vi "Register State.vi"() -> ()   [LabVIEW 2017]
uses:
  user.lib/_NEVSTOP/Communicable State Machine(CSM)/AdvanceAPI/CSM - Revert Arguments-Safe String.vi
  user.lib/_NEVSTOP/Communicable State Machine(CSM)/AdvanceAPI/CSM - Make String Arguments Safe.vi
  user.lib/_NEVSTOP/Communicable State Machine(CSM)/AdvanceAPI/CSM - Break Down Multiple States String.vi
  user.lib/_NEVSTOP/Communicable State Machine(CSM)/AdvanceAPI/CSM - Compact Multiple States.vi
  user.lib/_NEVSTOP/Communicable State Machine(CSM)/AdvanceAPI/CSM - Keywords.vi
  user.lib/_NEVSTOP/Communicable State Machine(CSM)/_Shared/Trim Single-line Text.vi
  user.lib/_NEVSTOP/Communicable State Machine(CSM)/Communicable State Machine.lvlib
panel:
  in  "API: API2 -@submodule2":bool
  in  "API: API1 -@submodule1":bool
  out "State History":string
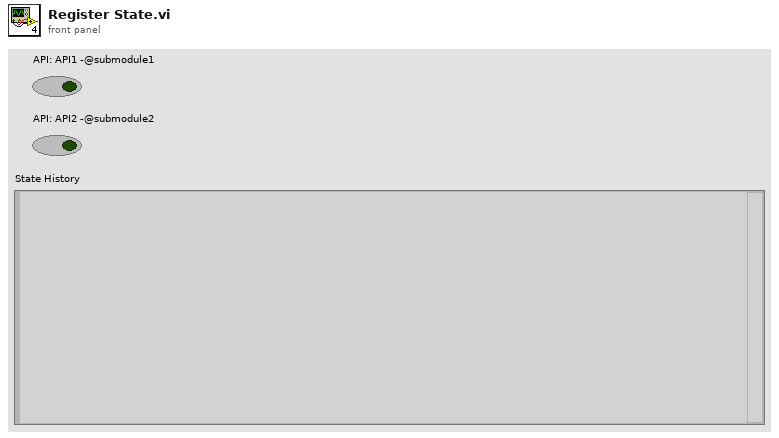
[diagram p1: front panel]
types:
  T1 = enum32{"Invalid", "Standard", "Closed", "Hidden", "Minimized", "Maximized"}
  T2 = enum32{"invalid app kind", "Development System", "Run Time System", "Student Edition", "Embedded LabVIEW", "Evaluation", "Custom"}
  T3 = typedef "Communicable State Machine.lvlib/_CSM_Response Source Message.ctl" = cluster{"‘State":string, "’Arguments":string, "’Error":errorcluster}
  T4 = cluster{"Current VI Reference":refnum<vi>, "Close Panel on Exit?":bool}
  T5 = cluster{"Core":cluster{"Current VI Reference":refnum<vi>, "Close Panel on Exit?":bool}, "Your Boolean data":bool, "Your string data":string}
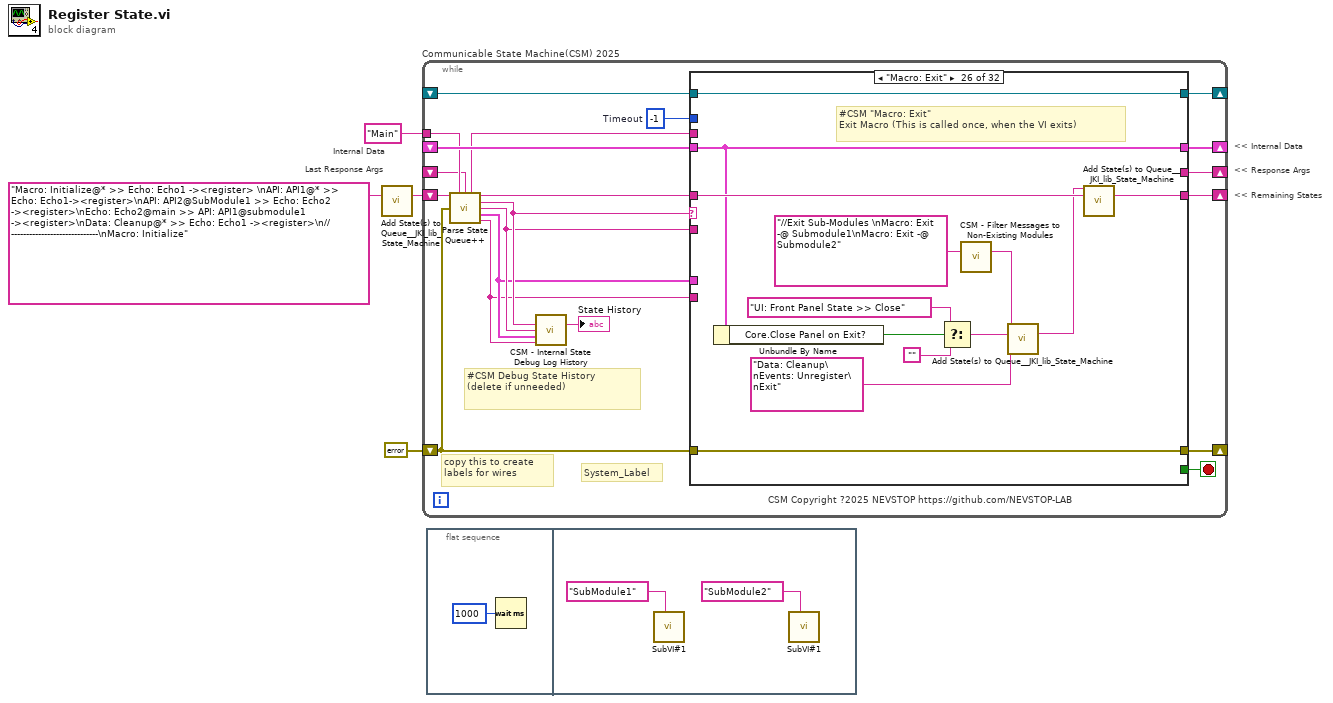
[diagram p0: block diagram]
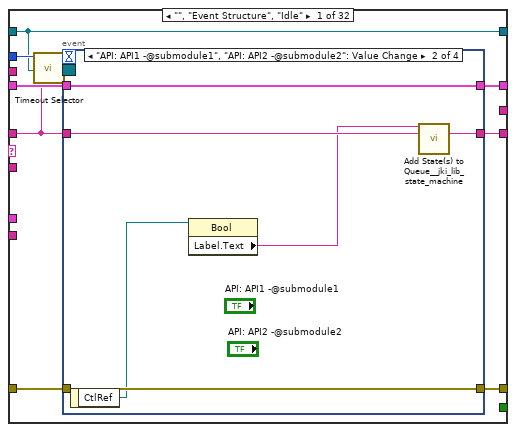
[diagram p2: hidden frame]
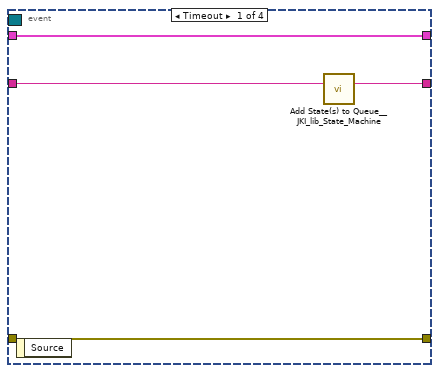
[diagram p3: hidden frame]
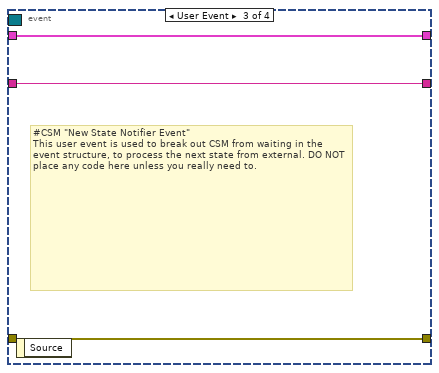
[diagram p4: hidden frame]
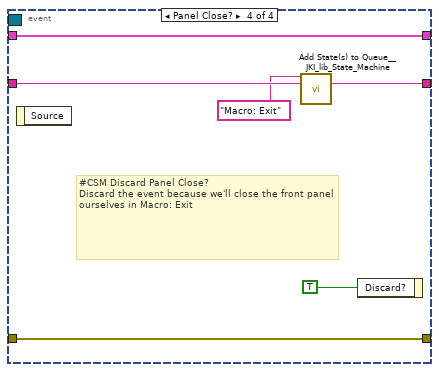
[diagram p5: hidden frame]
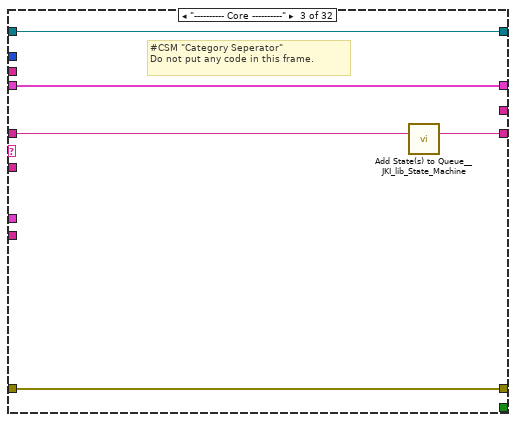
[diagram p7: hidden frame]
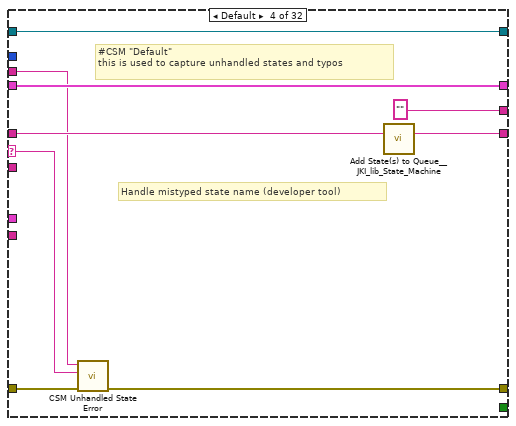
[diagram p8: hidden frame]
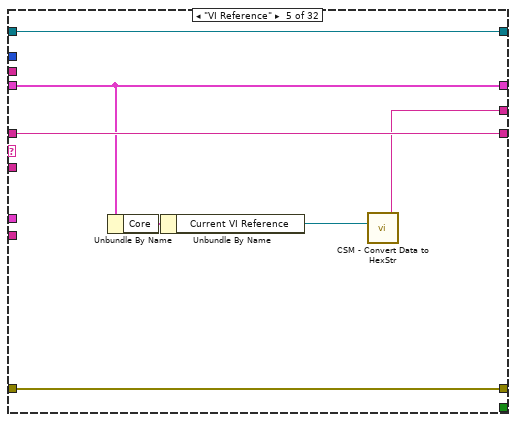
[diagram p9: hidden frame]
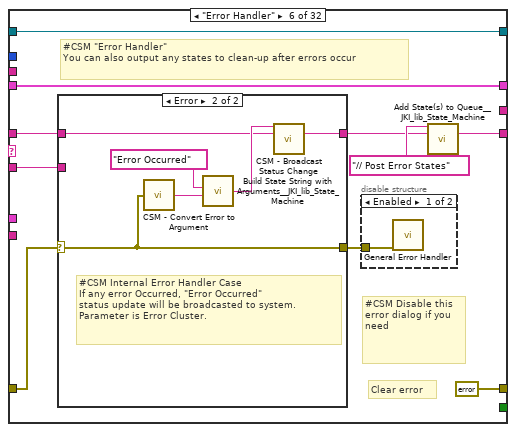
[diagram p10: hidden frame]
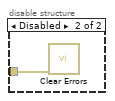
[diagram p11: hidden frame]
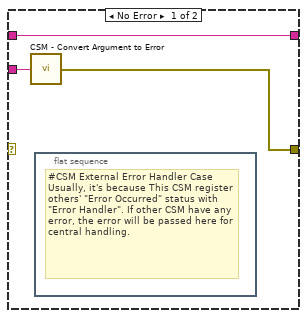
[diagram p12: hidden frame]
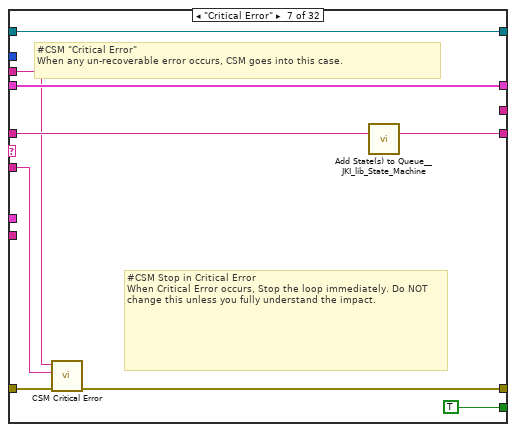
[diagram p13: hidden frame]
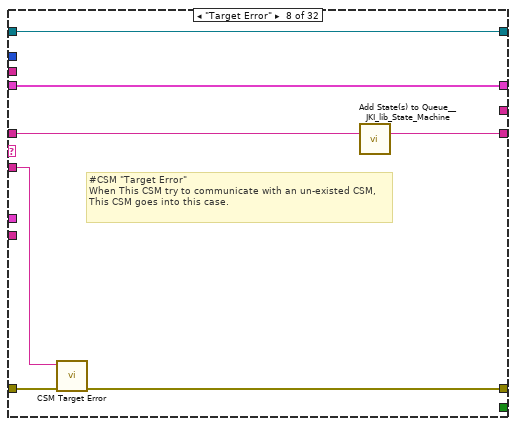
[diagram p14: hidden frame]
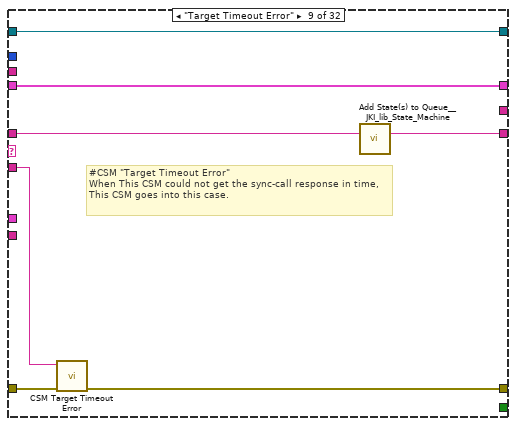
[diagram p15: hidden frame]
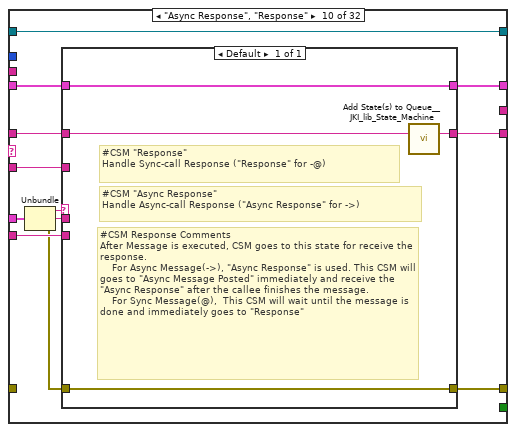
[diagram p16: hidden frame]
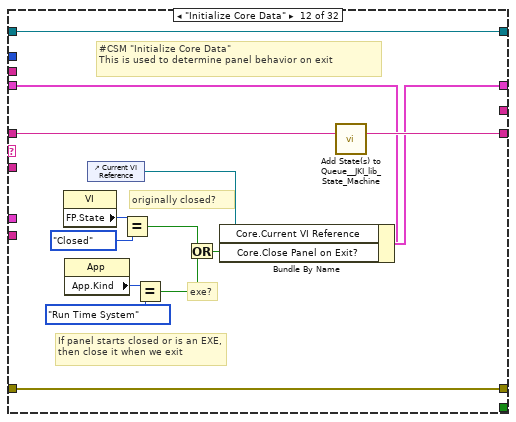
[diagram p18: hidden frame]
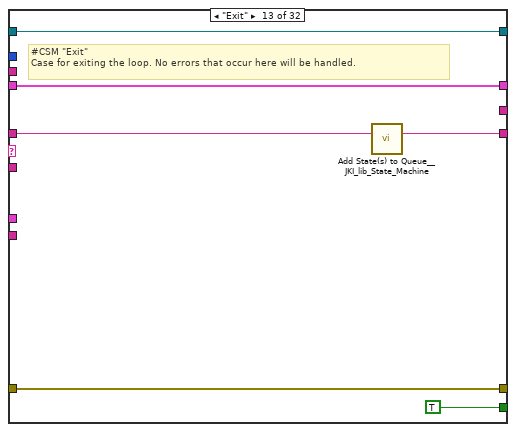
[diagram p19: hidden frame]
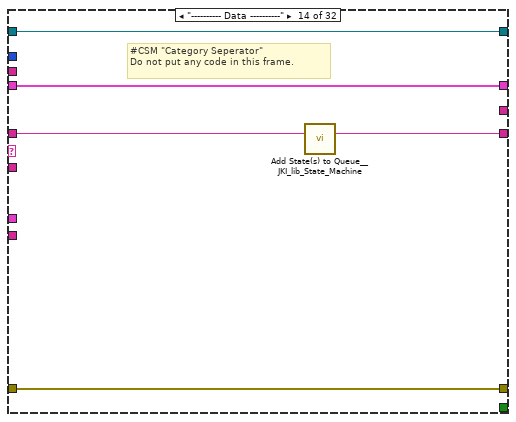
[diagram p20: hidden frame]
diagram:
  # "Last Response Args"
  # "Internal Data"
  # "<< Internal Data"
  # "<< Response Args"
  # "<< Remaining States"
  n1 = call <vilib>:"Add State(s) to Queue__JKI_lib_State_Machine.vi"("State(s) in (\"\")"="Macro: Initialize@* >> Echo: Echo1 -><register> \nAPI: API1@* >> Echo: Echo1-><register>\nAPI: API2@SubModule1 >> Echo: Echo2 -><register>\nEcho: Echo2@main >> API: API1@submodule1 -><register>\nData: Cleanup@* >> Echo: Echo1 -><register>\n//-----------------------------\nMacro: Initialize" ("Init State(\"Macro: Initialize\")")) -> ("States Out"=w4:string)  [unwired: 14 in]
  n2 = while "Communicable State Machine(CSM) 2025" {
    shift-right: [w19] -> _
    shift-left: _ -> [w18]
    shift-right: [w22] -> _
    shift-left: errorcluster {"status"=FALSE, "code"=0, "source"=""} ("error out") -> [w16]
    shift-right: [w21] -> _
    shift-left: w4 -> [w23]
    tunnel: "Main" ("Name(\"\" to use uuid)") -> [w12]
    shift-right: [w15] -> _
    shift-left: _ -> [w6]
    shift-right: [w14] -> _
    shift-left: _ -> [w13]
    stop <- w20 stop-if-true
    w17 = -1  # Timeout
    # "#CSM Debug State History\n(delete if unneeded)"
    # "copy this to create labels for wires"
    # "System_Label"
    # "CSM Copyright ?2025 NEVSTOP https://github.com/NEVSTOP-LAB"
    n3 = call "Parse State Queue++.vi"("State Queue"=w23, "Name(\"\" to use uuid)"=w12, "Response Arguments"=w6, "Previous Error"=w16) -> ("Name Used"=w7:string, "Remaining States"=w24:string, "Current State"=w11:string, "Arguments"=w10:string, ">> Response Source Message >>"=w9:T3, ">> Source CSM >>"=w8:string)  [unwired: 6 in]
    n4 = call "CSM - Internal State Debug Log History.vi"("State"=w11, "Arguments (\"\")"=w10, ">> Response Source Message >>"=w9, "Source (\"\")"=w8) -> ("Debug Log"=→"State History":string)  [unwired: 11 in]
    n5 = case shown="\"Macro: Exit\"" w11 {
      selector: w11 -> [_ _ _ w64 _ _ _ _ _ _ _ _ _ _ _ _ _ _ _ _ _ _ _ _ _ _ _ _ _ _ _ _]
      tunnel: w24 -> [w25 w55 w61 w69 w76 w82 w105 w111 w118 w127 w140 w155 w161 w166 w174 w181 w186 w193 w197 w203 w208 w215 w231 w301 w307 w320 w323 w328 w334 w342 w349 w354]
      tunnel: w10 -> [_ _ _ _ _ w81 w100 w110 w117 w126 _ _ _ _ _ _ _ _ _ _ _ w210 w225 _ _ _ _ _ w331 _ w343 _]
      tunnel: w18 -> [w32 w54 w58 w67 w75 w86 w106 w113 w120 w129 w139 w148 w159 w163 _ w176 w183 w192 w196 w200 w206 w213 w227 w298 w304 w317 w322 w327 w333 w339 w346 w351]
      tunnel: [w31 w56 w59 w62 w77 errorcluster {"status"=FALSE, "code"=0, "source"=""} ("error out") w101 w108 w115 w132 w141 w152 w158 w164 w171 w177 w184 w187 w195 w201 w205 w211 w228 w299 w305 w318 w324 w329 w335 w340 w347 w352] -> w22
      tunnel: w16 -> [w30 w56 w59 w70 w77 w83 w107 w109 w116 _ w141 w152 w158 w164 w171 w178 w184 _ w198 w201 w205 w212 w229 w299 w305 w318 w324 w329 w335 w340 w347 w352]
      tunnel: [w33 w55 w60 w68 w76 w78 w104 w114 w121 w128 w140 w154 w160 w165 w173 w180 w185 w193 w197 w202 w207 w214 w230 w300 w306 w319 w323 w328 w334 w341 w348 w353] -> w21
      tunnel: [_ _ _ _ _ _ TRUE _ _ _ _ _ TRUE _ _ _ _ _ _ _ _ _ _ _ _ _ _ _ _ _ _ _] -> w20
      tunnel: [w29 w54 w58 w67 w75 w86 w106 w113 w120 w130 w139 w153 w159 w163 w172 w176 w183 w192 w196 w200 w206 w213 w227 w298 w304 w317 w322 w327 w333 w339 w346 w351] -> w19
      tunnel: w17 -> [w28 _ _ _ _ _ _ _ _ _ _ _ _ _ _ _ _ _ _ _ _ _ _ _ _ _ _ _ _ _ _ _]
      tunnel: w8 -> [_ _ _ _ _ _ _ _ _ w124 _ _ _ _ _ _ _ _ _ _ _ _ _ _ _ _ _ _ _ _ w344 _]
      tunnel: w9 -> [_ _ _ _ _ _ _ _ _ w131 _ _ _ _ _ _ _ _ _ _ _ _ _ _ _ _ _ _ _ _ _ _]
      tunnel: [_ _ _ "" w71 _ _ _ _ _ _ _ _ _ _ _ _ _ _ _ _ _ _ _ _ _ _ "API1 Response" w330 _ _ _] -> w15
      tunnel: [w27 w53 w57 w65 w74 w85 w102 w112 w119 w133 w138 w142 w156 w162 w167 w175 w182 w191 w194 w199 w204 w209 w224 w297 w302 w310 w321 w326 w332 w338 w345 w350] -> w14
      tunnel: w13 -> [w27 w53 w57 w65 w74 w85 w102 w112 w119 w133 w138 w142 w156 w162 w167 w175 w182 _ w194 w199 w204 w209 w224 w297 w302 w310 w321 w326 w332 w338 w345 w350]
      tunnel: w7 -> [_ _ _ w63 _ _ w99 _ _ _ _ _ _ _ _ _ _ w190 _ _ _ _ _ _ _ _ _ _ _ _ _ _]
      frame "", "Event Structure", "Idle" {
        n6 = call "Timeout Selector.vi"("Remaining States"=w25, "Timeout Expected"=w28) -> ("Timeout"=w26:i32)  [unwired: 5 in]
        n7 = event shown="[1] \"API: API1 -@submodule1\", \"API: API2 -@submodule2\": Value Change" {
          selector: w27 -> [_ _ _ _]
          dyn-events: _ -> [_ _ _ _]
          timeout: w26 -> [_ _ _ _]
          tunnel: w25 -> [w37 w40 w45 w52]
          tunnel: [w36 w41 w45 w51] -> w33
          tunnel: w32 -> [w34 w42 w46 w49]
          tunnel: [w35 w43 w44 w50] -> w31
          tunnel: w30 -> [w35 w43 w44 w50]
          tunnel: [w34 w42 w46 w49] -> w29
          event Timeout {
            n8 = event-data() -> ()  [unwired: 1 in, 1 out]
            n9 = call <vilib>:"Add State(s) to Queue__JKI_lib_State_Machine.vi"("State(s) in (\"\")"=w37) -> ("States Out"=w36:string)  [unwired: 14 in]
          }
          event "API: API1 -@submodule1", "API: API2 -@submodule2": Value Change {
            n10 = event-data() -> ("CtlRef"=w39:refnum<vi>)  [unwired: 1 in]
            n11 = property class="Bool"(reference=w39) -> ("Label.Text"=w38:string)  [unwired: 1 in, 2 out]
            n12 = call <vilib>:"Add State(s) to Queue__jki_lib_state_machine.vi"("State(s) in Front (\"\")"=w38, "State(s) in (\"\")"=w40) -> ("States Out"=w41:string)  [unwired: 13 in]
          }
          event User Event {
            # "#CSM \"New State Notifier Event\"\nThis user event is used to break out CSM from waiting in the event structure, to process the next state from external. DO NOT place any code here unless you really need to."
            n13 = event-data() -> ()  [unwired: 1 in, 1 out]
          }
          event Panel Close? {
            # "#CSM Discard Panel Close?\nDiscard the event because we'll close the front panel ourselves in Macro: Exit"
            n14 = event-data() -> ()  [unwired: 1 in, 1 out]
            n15 = call <vilib>:"Add State(s) to Queue__JKI_lib_State_Machine.vi"("State(s) in Front (\"\")"="Macro: Exit", "State(s) in (\"\")"=w52) -> ("States Out"=w51:string)  [unwired: 13 in]
            n16 = event-data("Discard?"=TRUE) -> ()  [unwired: 1 in, 1 out]
          }
        }
      }
      frame "CSM Documentation" {
        # "#CSM README FIRST\n\nCommunicable State Machine(CSM) is a LabVIEW application framework that builds upon JKI State Machine(JKISM). It follows the pattern of JKISM and extends the keywords to describe message communication between modules, including concepts such as Sync-Message, Async-Message, Subscription/Unsubscription of status - essential elements for creating reusable code modules. For more information, please visit the CSM wiki: https://nevstop-lab.github.io/CSM-Wiki/\n\nFor instructions on JKI State Machine, visit: http://jki.net/state-machine/\nFor information about CSM, visit: https://github.com/NEVSTOP-LAB"
        # "#CSM \"Documentation\"\nCase for holding CSM Documenation"
      }
      frame "---------- Core ----------" {
        # "#CSM \"Category Seperator\"\nDo not put any code in this frame."
        n17 = call <vilib>:"Add State(s) to Queue__JKI_lib_State_Machine.vi"("State(s) in (\"\")"=w61) -> ("States Out"=w60:string)  [unwired: 14 in]
      }
      frame Default {
        # "#CSM \"Default\"\nthis is used to capture unhandled states and typos"
        # "Handle mistyped state name (developer tool)"
        n18 = call "CSM Unhandled State Error.vi"("error in (no error)"=w70, "Current State"=w64, "CSM Name"=w63) -> ("error out"=w62:errorcluster)  [unwired: 8 in]
        n19 = call <vilib>:"Add State(s) to Queue__JKI_lib_State_Machine.vi"("State(s) in (\"\")"=w69) -> ("States Out"=w68:string)  [unwired: 14 in]
      }
      frame "VI Reference" {
        n20 = Unbundle By Name(w75) -> ("Core"=w73:T4)
        n21 = Unbundle By Name(w73) -> ("Current VI Reference"=w72:refnum<vi>)
        n22 = call "CSM - Convert Data to HexStr.vi"("Variant"=w72) -> ("HEX String (0-9,A-F)"=w71:string)  [unwired: 8 in]
      }
      frame "Error Handler" {
        # "#CSM Disable this error dialog if you need"
        # "#CSM \"Error Handler\"\nYou can also output any states to clean-up after errors occur"
        # "Clear error"
        n23 = case shown="Error" w83 {
          selector: w83 -> [_ w93]
          tunnel: [w92 w95] -> w79
          tunnel: w82 -> [w92 w94]
          tunnel: w81 -> [w91 _]
          tunnel: [w90 w93] -> w84
          frame No Error {
            n24 = call "CSM - Convert Argument to Error.vi"("Argument"=w91) -> ("error"=w90:errorcluster)  [unwired: 4 in]
            n25 = flat-sequence {
              frame #0 {
                # "#CSM External Error Handler Case\nUsually, it's because This CSM register others' \"Error Occurred\" status with \"Error Handler\". If other CSM have any error, the error will be passed here for central handling."
              }
            }
          }
          frame Error {
            # "#CSM Internal Error Handler Case \nIf any error Occurred, \"Error Occurred\" \nstatus update will be broadcasted to system.\nParameter is Error Cluster."
            n26 = call "CSM - Convert Error to Argument.vi"("error"=w93) -> ("Argument"=w97:string)  [unwired: 4 in]
            n27 = call <vilib>:"Build State String with Arguments__JKI_lib_State_Machine.vi"("Arguments (\"\")"=w97, "State"="Error Occurred" ("Status with Arguments")) -> ("State with Arguments"=w96:string)  [unwired: 4 in]
            n28 = call "CSM - Broadcast Status Change.vi"("Status with Arguments"=w96, "State Queue"=w94) -> ("Remaining States"=w95:string)  [unwired: 13 in]
          }
        }
        n29 = disable-structure shown="Enabled" {
          disable-tunnel: w84 -> [w88 w89]
          frame Enabled {
            n30 = call <vilib>:"General Error Handler.vi"("error in (no error)"=w88) -> ()  [unwired: 10 in, 5 out]
          }
          frame Disabled {
            n31 = call <vilib>:"Clear Errors.vi"("error in (no error)"=w89) -> ()  [unwired: 5 in, 2 out]
          }
        }
        n32 = call <vilib>:"Add State(s) to Queue__JKI_lib_State_Machine.vi"("State(s) in Front (\"\")"="// Post Error States", "State(s) in (\"\")"=w79) -> ("States Out"=w78:string)  [unwired: 13 in]
      }
      frame "Critical Error" {
        # "#CSM Stop in Critical Error\nWhen Critical Error occurs, Stop the loop immediately. Do NOT change this unless you fully understand the impact."
        # "#CSM \"Critical Error\"\nWhen any un-recoverable error occurs, CSM goes into this case."
        n33 = call "CSM Critical Error.vi"("error in (no error)"=w107, "Arugments(as Reason)"=w100, "CSM Name"=w99) -> ("error out"=w101:errorcluster)  [unwired: 8 in]
        n34 = call <vilib>:"Add State(s) to Queue__JKI_lib_State_Machine.vi"("State(s) in (\"\")"=w105) -> ("States Out"=w104:string)  [unwired: 14 in]
      }
      frame "Target Error" {
        # "#CSM \"Target Error\"\nWhen This CSM try to communicate with an un-existed CSM, This CSM goes into this case."
        n35 = call "CSM Target Error.vi"("error in (no error)"=w109, "Arguments(as CSM Name)"=w110) -> ("error out"=w108:errorcluster)  [unwired: 9 in]
        n36 = call <vilib>:"Add State(s) to Queue__JKI_lib_State_Machine.vi"("State(s) in (\"\")"=w111) -> ("States Out"=w114:string)  [unwired: 14 in]
      }
      frame "Target Timeout Error" {
        # "#CSM \"Target Timeout Error\"\nWhen This CSM could not get the sync-call response in time, This CSM goes into this case."
        n37 = call "CSM Target Timeout Error.vi"("error in (no error)"=w116, "Arguments(as CSM Name)"=w117) -> ("error out"=w115:errorcluster)  [unwired: 9 in]
        n38 = call <vilib>:"Add State(s) to Queue__JKI_lib_State_Machine.vi"("State(s) in (\"\")"=w118) -> ("States Out"=w121:string)  [unwired: 14 in]
      }
      frame "Async Response", "Response" {
        n39 = Unbundle(w131) -> ("‘State"=w125:string, "’Arguments"=w123:string, "’Error"=w122:errorcluster)
        n40 = case shown="Default" w125 {
          tunnel: [w137] -> w132
          tunnel: w122 -> [w137]
          tunnel: [w136] -> w130
          tunnel: w129 -> [w136]
          tunnel: [w134] -> w128
          tunnel: w127 -> [w135]
          tunnel: w126 -> [_]
          tunnel: w124 -> [_]
          tunnel: w123 -> [_]
          frame Default {
            # "#CSM Response Comments\nAfter Message is executed, CSM goes to this state for receive the response.\n    For Async Message(->), \"Async Response\" is used. This CSM will goes to \"Async Message Posted\" immediately and receive the \"Async Response\" after the callee finishes the message.\n    For Sync Message(@),  This CSM will wait until the message is done and immediately goes to \"Response\""
            # "#CSM \"Async Response\"\nHandle Async-call Response (\"Async Response\" for ->)"
            # "#CSM \"Response\"\nHandle Sync-call Response (\"Response\" for -@)"
            n41 = call <vilib>:"Add State(s) to Queue__JKI_lib_State_Machine.vi"("State(s) in (\"\")"=w135) -> ("States Out"=w134:string)  [unwired: 14 in]
          }
        }
      }
      frame "Async Message Posted" {
        # "#CSM \"Async Message Posted\"\nAfter Async Message is posted (-> or ->| ), CSM goes to this state for post-action.\nYou can use Argument - State to tell which Async Message is called."
      }
      frame "Initialize Core Data" {
        # "#CSM \"Initialize Core Data\"\nThis is used to determine panel behavior on exit"
        # "originally closed?"
        # "exe?"
        # "If panel starts closed or is an EXE, then close it when we exit"
        n42 = property class="VI"() -> ("FP.State"=w145:T1)  [unwired: 2 in, 2 out]
        n43 = property class="App"() -> ("App.Kind"=w151:T2)  [unwired: 2 in, 2 out]
        n44 = control-ref of="Current VI Reference"() -> (w146:refnum<vi>)
        n45 = Equal?(x=w145, y=T1."Closed" ("Front Panel Window:State")) -> (x = y?=w143:bool)
        n46 = Equal?(x=w151, y=T2."Run Time System" ("Application:Kind")) -> (x = y?=w149:bool)
        n47 = Or(x=w143, y=w149) -> (x .or. y?=w147:bool)
        n48 = Bundle By Name(cluster=w148, "Core.Current VI Reference"=w146, "Core.Close Panel on Exit?"=w147) -> (w153:T5)
        n49 = call <vilib>:"Add State(s) to Queue__JKI_lib_State_Machine.vi"("State(s) in (\"\")"=w155) -> ("States Out"=w154:string)  [unwired: 14 in]
      }
      frame "Exit" {
        # "#CSM \"Exit\"\nCase for exiting the loop. No errors that occur here will be handled."
        n50 = call <vilib>:"Add State(s) to Queue__JKI_lib_State_Machine.vi"("State(s) in (\"\")"=w161) -> ("States Out"=w160:string)  [unwired: 14 in]
      }
      frame "---------- Data ----------" {
        # "#CSM \"Category Seperator\"\nDo not put any code in this frame."
        n51 = call <vilib>:"Add State(s) to Queue__JKI_lib_State_Machine.vi"("State(s) in (\"\")"=w166) -> ("States Out"=w165:string)  [unwired: 14 in]
      }
      frame "Data: Initialize" {
        w168 = T4 {"Current VI Reference"=refnum, "Close Panel on Exit?"=FALSE}  # Core
        w170 = TRUE  # Your Boolean data
        w169 = ""  # Your string data
        # "#CSM do not delete - used by framework"
        # "#CSM Expand Bundle to add new data elements to shift register data."
        # "#CSM Add new data here."
        # "Initialize the shift-register data, here.\n(data names are defined by what you wire into the bundle function)"
        n52 = Bundle("Core"=w168, "Your Boolean data"=w170, "Your string data"=w169) -> (w172:T5)  [unwired: 1 in]
        n53 = call <vilib>:"Add State(s) to Queue__JKI_lib_State_Machine.vi"("State(s) in (\"\")"=w174) -> ("States Out"=w173:string)  [unwired: 14 in]
      }
      frame "Data: Cleanup" {
        # "Cleanup any data and references, here.\n(this is called automatically, by the Macro: Exit)"
        n54 = Unbundle By Name(w176) -> ("Core.Current VI Reference"=w179:refnum<vi>)
        n55 = Close Reference(reference=w179, error in (no error)=w178) -> (error out=w177:errorcluster)
        n56 = call <vilib>:"Add State(s) to Queue__JKI_lib_State_Machine.vi"("State(s) in (\"\")"=w181) -> ("States Out"=w180:string)  [unwired: 14 in]
      }
      frame "---------- Events ----------" {
        # "#CSM \"Category Seperator\"\nDo not put any code in this frame."
        n57 = call <vilib>:"Add State(s) to Queue__JKI_lib_State_Machine.vi"("State(s) in (\"\")"=w186) -> ("States Out"=w185:string)  [unwired: 14 in]
      }
      frame "Events: Register" {
        # "#CSM \"Events: Register\"\nRegister user event. New Message Event is registered to break CSM waiting in event structure by default."
        # "#CSM Register New Message Event\nRegister message event to break Waiting in Event structure."
        n58 = call "CSM - Get New State Notifier Event.vi"("Name(\"\" to use uuid) in"=w190) -> ("Error out"=w188:errorcluster, "New State Notifier Event"=w189:refnum<user-event>)  [unwired: 9 in]
        n59 = register-events(error in=w188, w189) -> (reference out=w191:refnum<event-registration>, error out=w187:errorcluster)  [unwired: 1 in]
      }
      frame "Events: Unregister" {
        # "#CSM \"Events: Unregister\"\nUnregister user event."
        n60 = Unregister For Events(event registration refnum=w194, error in=w198) -> (error out=w195:errorcluster)
      }
      frame "---------- UI ----------" {
        # "#CSM \"Category Seperator\"\nDo not put any code in this frame."
        n61 = call <vilib>:"Add State(s) to Queue__JKI_lib_State_Machine.vi"("State(s) in (\"\")"=w203) -> ("States Out"=w202:string)  [unwired: 14 in]
      }
      frame "UI: Initialize" {
        # "#CSM \"UI: Initialize\"\nInitialize the User Interface, here.\n(this is called automatically, by the Macro: Init)"
        n62 = call <vilib>:"Add State(s) to Queue__JKI_lib_State_Machine.vi"("State(s) in (\"\")"=w208) -> ("States Out"=w207:string)  [unwired: 14 in]
      }
      frame "UI: Cursor Set" {
        # "#CSM \"UI: Cursor Set\"\nSet and Unset Cursor Busy.\n(Usage: \"UI: Cursor Set >> Busy|Idle\")"
        # "Argument"
        n63 = disable-structure shown="Default" {
          disable-tunnel: w212 -> [w218 w223]
          disable-tunnel: [w217 w223] -> w211
          disable-tunnel: w210 -> [w216 _]
          frame condition #0 (active) {
            n64 = case shown="\"Idle\", Default" w216 {
              tunnel: w218 -> [w220 w222]
              tunnel: [w219 w221] -> w217
              frame "Idle", Default {
                n65 = call <vilib>:"Unset Busy.vi"("error in (no error)"=w220) -> ("error out"=w219:errorcluster)  [unwired: 10 in]
              }
              frame "Busy" {
                n66 = call <vilib>:"Set Busy.vi"("error in (no error)"=w222) -> ("error out"=w221:errorcluster)  [unwired: 9 in, 1 out]
              }
            }
          }
          frame condition #1 {
          }
        }
        n67 = call <vilib>:"Add State(s) to Queue__JKI_lib_State_Machine.vi"("State(s) in (\"\")"=w215) -> ("States Out"=w214:string)  [unwired: 14 in]
      }
      frame "UI: Front Panel State" {
        # "#CSM \"UI: Front Panel State\"\nSet Front Panel Open or Closed\n(Usage: \"UI: Front Panel State >> Open|Close\")"
        # "Argument"
        n68 = Unbundle By Name(w227) -> ("Core.Current VI Reference"=w226:refnum<vi>)
        n69 = call <vilib>:"Add State(s) to Queue__JKI_lib_State_Machine.vi"("State(s) in (\"\")"=w231) -> ("States Out"=w230:string)  [unwired: 14 in]
        n70 = case shown="\"Close\", \"Closed\"" w225 {
          tunnel: w229 -> [w237 w252 w263 w276 w289]
          tunnel: [w239 w253 w265 w278 w291] -> w228
          tunnel: w226 -> [w238 w250 w264 w277 w290]
          frame "Open", "Standard", Default {
            w232 = T1."Standard" ("State")
            n71 = property class="VI"(reference=w238, error in=w237) -> (reference out=w235:refnum<vi>, error out=w236:errorcluster, "FP.State"=w234:T1)
            n72 = Not Equal?(x=w234, y=w232) -> (x != y?=w233:bool)
            n73 = case shown="True" w233 {
              tunnel: [w243 w245] -> w239
              tunnel: w236 -> [w242 w245]
              tunnel: w235 -> [w241 _]
              tunnel: w232 -> [w240 _]
              frame True {
                n74 = invoke class="VI" method="FP.Open"(reference=w241, error in=w242, "Activate"=TRUE, "State"=w240) -> (error out=w243:errorcluster)  [unwired: 1 in, 4 out]
              }
              frame False {
              }
            }
          }
          frame "Close", "Closed" {
            n75 = property class="VI"(reference=w250, error in=w252) -> (reference out=w249:refnum<vi>, error out=w251:errorcluster, "FP.State"=w247:T1)
            n76 = Not Equal?(x=w247, y=T1."Closed" ("Front Panel Window:State")) -> (x != y?=w246:bool)
            n77 = case shown="False" w246 {
              tunnel: [w254 w257] -> w253
              tunnel: w251 -> [w254 w256]
              tunnel: w249 -> [_ w255]
              frame False {
              }
              frame True {
                n78 = invoke class="VI" method="FP.Close"(reference=w255, error in=w256) -> (error out=w257:errorcluster)  [unwired: 1 in, 2 out]
              }
            }
          }
          frame "Hidden", "Hide" {
            w258 = T1."Hidden" ("State")
            n79 = property class="VI"(reference=w264, error in=w263) -> (reference out=w261:refnum<vi>, error out=w262:errorcluster, "FP.State"=w260:T1)
            n80 = Not Equal?(x=w260, y=w258) -> (x != y?=w259:bool)
            n81 = case shown="True" w259 {
              tunnel: [w269 w270] -> w265
              tunnel: w262 -> [w268 w270]
              tunnel: w261 -> [w267 _]
              tunnel: w258 -> [w266 _]
              frame True {
                n82 = invoke class="VI" method="FP.Open"(reference=w267, error in=w268, "State"=w266) -> (error out=w269:errorcluster)  [unwired: 2 in, 4 out]
              }
              frame False {
              }
            }
          }
          frame "Minimize", "Minimized" {
            w271 = T1."Minimized" ("State")
            n83 = property class="VI"(reference=w277, error in=w276) -> (reference out=w274:refnum<vi>, error out=w275:errorcluster, "FP.State"=w273:T1)
            n84 = Not Equal?(x=w273, y=w271) -> (x != y?=w272:bool)
            n85 = case shown="True" w272 {
              tunnel: [w282 w283] -> w278
              tunnel: w275 -> [w281 w283]
              tunnel: w274 -> [w280 _]
              tunnel: w271 -> [w279 _]
              frame True {
                n86 = invoke class="VI" method="FP.Open"(reference=w280, error in=w281, "State"=w279) -> (error out=w282:errorcluster)  [unwired: 2 in, 4 out]
              }
              frame False {
              }
            }
          }
          frame "Maximize", "Maximized" {
            w284 = T1."Maximized" ("State")
            n87 = property class="VI"(reference=w290, error in=w289) -> (reference out=w287:refnum<vi>, error out=w288:errorcluster, "FP.State"=w286:T1)
            n88 = Not Equal?(x=w286, y=w284) -> (x != y?=w285:bool)
            n89 = case shown="True" w285 {
              tunnel: [w295 w296] -> w291
              tunnel: w288 -> [w294 w296]
              tunnel: w287 -> [w293 _]
              tunnel: w284 -> [w292 _]
              frame True {
                n90 = invoke class="VI" method="FP.Open"(reference=w293, error in=w294, "State"=w292) -> (error out=w295:errorcluster)  [unwired: 2 in, 4 out]
              }
              frame False {
              }
            }
          }
        }
      }
      frame "---------- Macro ----------" {
        # "#CSM \"Category Seperator\"\nDo not put any code in this frame."
        n91 = call <vilib>:"Add State(s) to Queue__JKI_lib_State_Machine.vi"("State(s) in (\"\")"=w301) -> ("States Out"=w300:string)  [unwired: 14 in]
      }
      frame "Macro: Initialize" {
        w303 = "Data: Initialize\nInitialize Core Data\nEvents: Register\nUI: Initialize\nUI: Front Panel State >> Open"  # Data: Initialize Initialize Core Data Events: Register UI: Initialize UI: Front Panel State >> Open
        # "#CSM \"Macro: Initialize\"\nInitialization Macro (This is called once, when the VI starts)"
        n92 = call <vilib>:"Add State(s) to Queue__JKI_lib_State_Machine.vi"("State(s) in Front (\"\")"=w303, "State(s) in (\"\")"=w307) -> ("States Out"=w306:string)  [unwired: 13 in]
      }
      frame "Macro: Exit" {
        # "#CSM \"Macro: Exit\"\nExit Macro (This is called once, when the VI exits)"
        n93 = Unbundle By Name(w317) -> ("Core.Close Panel on Exit?"=w316:bool)
        n94 = Select(t="UI: Front Panel State >> Close", s=w316, f="") -> (s? t:f=w313:string)
        n95 = call "CSM - Filter Messages to Non-Existing Modules.vi"("State(s) in (\"\")"="//Exit Sub-Modules \nMacro: Exit -@ Submodule1\nMacro: Exit -@ Submodule2") -> ("States Out"=w308:string)  [unwired: 14 in]
        n96 = call <vilib>:"Add State(s) to Queue__JKI_lib_State_Machine.vi"("State(s) in Front (\"\")"=w308, "State(s) in (\"\")"=w313, "State(s) at Back (\"\")"="Data: Cleanup\nEvents: Unregister\nExit") -> ("States Out"=w311:string)  [unwired: 12 in]
        n97 = call <vilib>:"Add State(s) to Queue__JKI_lib_State_Machine.vi"("State(s) in Front (\"\")"=w311, "State(s) in (\"\")"=w320) -> ("States Out"=w319:string)  [unwired: 13 in]
      }
      frame "---------- API ----------" {
        # "#CSM \"Category Seperator\"\nDo not put any code in this frame."
      }
      frame "API: API1" {
        # "#CSM API Example\nCopy/Rename this case for your own API"
        # "#CSM Response\nConnect this to return the response of your API"
        # "#CSM >> Source CSM >>\nIf you need to tell who triggered this state , use this string. If it's this case itself, this string is \"\"."
        # "#CSM >> Arguments >>\nDeal with the parameter if any"
      }
      frame "API: API2" {
        # "#CSM API Example\nCopy/Rename this case for your own API"
        # "unpack Hex String  to Variant\nif complex parameter is needed."
        n98 = call "CSM - Convert HexStr to Data.vi"("HEX String"=w331) -> ()  [unwired: 7 in, 2 out]
        n99 = disable-structure shown="Disabled" {
          disable-tunnel: [w336 "API2 Response"] -> w330
          frame Disabled {
            # "pack variant to hexstr \nif complex response is needed."
            # "complex Response"
            n100 = call "CSM - Convert Data to HexStr.vi"() -> ("HEX String (0-9,A-F)"=w336:string)  [unwired: 9 in]
          }
          frame Enabled {
          }
        }
      }
      frame "---------- Action ----------" {
        # "#CSM \"Category Seperator\"\nDo not put any code in this frame."
        n101 = call <vilib>:"Add State(s) to Queue__JKI_lib_State_Machine.vi"("State(s) in (\"\")"=w342) -> ("States Out"=w341:string)  [unwired: 14 in]
      }
      frame "Echo: Echo1" {
        # "#CSM \"Internal State\"\nThis category is used for holding internal states"
        n102 = One Button Dialog(message=w344, button name ("OK")=w343) -> ()  [unwired: 1 out]
        n103 = call <vilib>:"Add State(s) to Queue__JKI_lib_State_Machine.vi"("State(s) in (\"\")"=w349) -> ("States Out"=w348:string)  [unwired: 14 in]
      }
      frame "Echo: Echo2" {
        # "#CSM \"Internal State\"\nThis category is used for holding internal states"
        n104 = call <vilib>:"Add State(s) to Queue__JKI_lib_State_Machine.vi"("State(s) in (\"\")"=w354) -> ("States Out"=w353:string)  [unwired: 14 in]
      }
    }
  }
  n105 = flat-sequence {
    frame #0 {
      n106 = Wait (ms)(milliseconds to wait=u32 1000) -> ()  [unwired: 1 out]
    }
    frame #1 {
      n107 = call "SubVI#1.vi"("Name(\"\" to use uuid)"="SubModule1" ("Name(\"\" to use uuid)")) -> ()  [unwired: 11 in]
      n108 = call "SubVI#1.vi"("Name(\"\" to use uuid)"="SubModule2" ("Name(\"\" to use uuid)")) -> ()  [unwired: 11 in]
    }
  }
